vi "waveTriangular.vi"(1 "smoothing param":dbl, 2 "w":dbl, 3 "t":dbl) -> (0 "y":dbl)   [LabVIEW 2017]
panel:
  # "https://mathematica.stackexchange.com/questions/38293/make-a-differentiable-smooth-sawtooth-waveform"
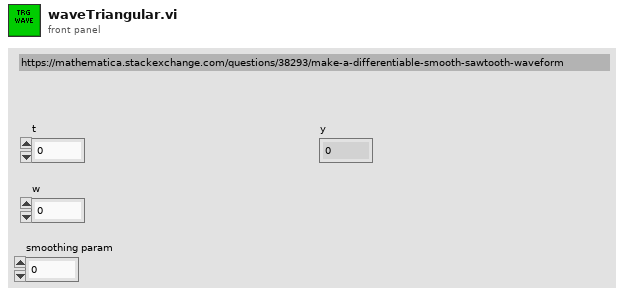
[diagram p1: front panel]
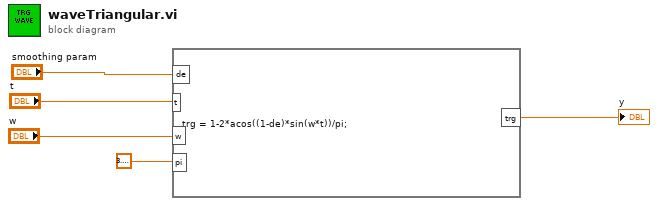
[diagram p0: block diagram]
diagram:
  n1 = formula code="trg = 1-2*acos((1-de)*sin(w*t))/pi;"("t"="t", "w"="w", "pi"=3.141592653589793, "de"="smoothing param") -> ("trg"=→"y":dbl)
